vi "To Engine Groups.vi"(9 "Type":T1(ring), 11 "Group":T4[](array[typedef])) -> (1 "Names":string[](array[string]), 3 "Engine Groups":T3(array[cluster]) {"VS Refs" format="%.0x"})   [LabVIEW 2015, in "Modbus Master System Explorer.lvlib"]
uses:
  Modbus Master System Explorer.lvlib
  Engine/SubVIs/Bulk Data Access.ctl
  Modbus Type.ctl
  Shared/Controls/Data Model/Channel.ctl
  <vilib>/NI Veristand/Custom Device API/Custom Device Channel Type.ctl
  Shared/Controls/Data Model/Mapping.ctl
  Shared/Controls/Data Model/DataType.ctl
  <vilib>/NI Veristand/Custom Device API/Custom Device Item Ref.ctl
  Shared/Modbus Master Shared.lvlib
  <vilib>/NI VeriStand/Custom Device API/Custom Device API.lvlib
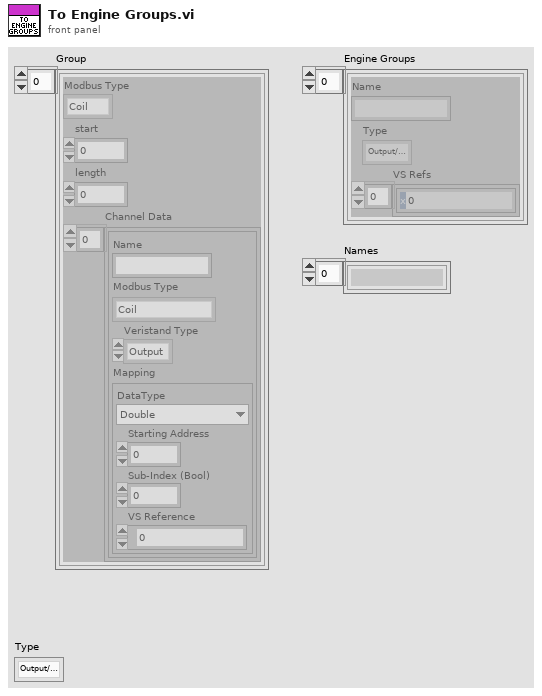
[diagram p1: front panel]
types:
  T1 = enum16{"Output/Write", "Input/Read", "Input/ReadWrite"}
  T2 = typedef "Custom Device API.lvlib/Custom Device Item Ref.ctl" = u64
  T3 = cluster{"Name":string, "Type":enum16{"Output/Write", "Input/Read", "Input/ReadWrite"}, "VS Refs":T2[]}[]
  T4 = typedef "Modbus Master Shared.lvlib/Bulk Data Access.ctl" = cluster{"Modbus Type":T5, "start":u16, "length":u16, "Channel Data":T6[]}
  T5 = typedef "Modbus Master Shared.lvlib/Modbus Type.ctl" = enum16{"Coil", "Discrete Input", "Holding Register", "Input Register"}
  T6 = typedef "Modbus Master Shared.lvlib/Channel.ctl" = cluster{"Name":string, "Modbus Type":T5, "Veristand Type":T7, "Mapping":T8}
  T7 = typedef "Custom Device API.lvlib/Custom Device Channel Type.ctl" = enum16{"Input", "Output"}
  T8 = typedef "Modbus Master Shared.lvlib/Mapping.ctl" = cluster{"DataType":T9, "Starting Address":u16, "Sub-Index (Bool)":u16, "VS Reference":T2}
  T9 = typedef "Modbus Master Shared.lvlib/DataType.ctl" = enum16{"Double", "Single", "I64", "I32", "I16", "I8", "U64", "U32", "U16", "U8", "Boolean"}
  T10 = cluster{"Name":string, "Type":enum16{"Output/Write", "Input/Read", "Input/ReadWrite"}, "VS Refs":T2[]}
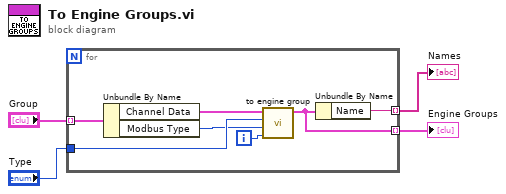
[diagram p0: block diagram]
diagram:
  n1 = for {
    tunnel: "Type" -> [w10]
    tunnel: [w7] -> w3 mode=indexing
    tunnel: "Group" -> [w9] mode=indexing
    tunnel: [w6] -> w1 mode=indexing
    i -> [w8]
    n2 = Unbundle By Name(w9) -> ("Channel Data"=w11:T6[], "Modbus Type"=w5:T5)
    n3 = call "to engine group.vi"("Index"=w8, "Modbus Type"=w5, "Access"=w10, "Channels"=w11) -> ("Group"=w7:T10)  [unwired: 7 in]
    n4 = Unbundle By Name(w7) -> ("Name"=w6:string)
  }
  "Engine Groups" <- w3
  "Names" <- w1
